vi "Control_sensors.vi"() -> ()   [LabVIEW 2019]
panel:
  out "output data":bool[](array[boolean])
  in  "Magneto (F) / Accelerometer (T)":bool
  in  "Stop":bool
  in  "Start":bool
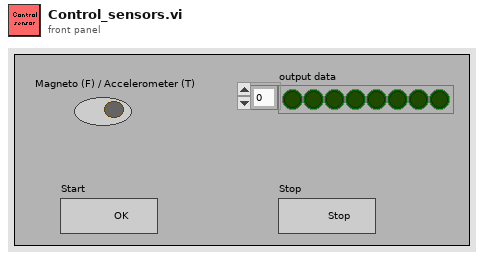
[diagram p1: front panel]
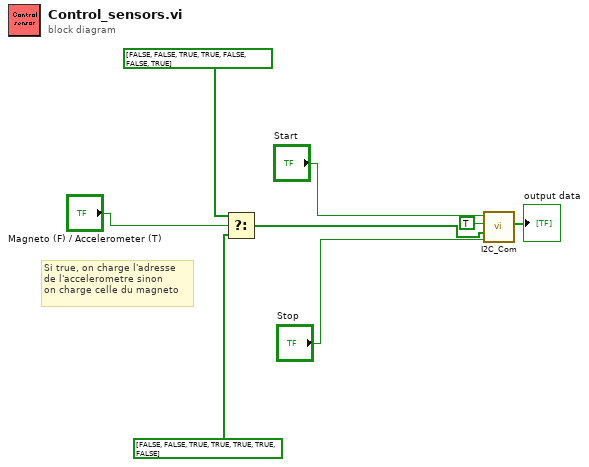
[diagram p0: block diagram]
diagram:
  # "Si true, on charge l'adresse\nde l'accelerometre sinon\non charge celle du magneto"
  n1 = Select(t=bool[] [FALSE, FALSE, TRUE, TRUE, FALSE, FALSE, TRUE], s="Magneto (F) / Accelerometer (T)", f=bool[] [FALSE, FALSE, TRUE, TRUE, TRUE, TRUE, FALSE]) -> (s? t:f=w5:bool[])
  n2 = call "I2C_Com.vi"("Stop"="Stop", "Address"=w5, "Read / Write"=TRUE, "Start"="Start") -> ("output data"=→"output data":bool[])  [unwired: 7 in]
